vi "Destroy.vi"(0 "reference in":refnum<class "Devices Controller.lvclass">, 5 "error in (no error)":errorcluster) -> (14 "reference out":refnum<class "Devices Controller.lvclass">, 19 "error out":errorcluster)   [LabVIEW 2015, in "Devices Controller.lvclass"]
doc: "Destructor."
uses:
  Devices Controller.lvclass
  <vilib>/addons/_AddQ/G#Object/G#Object.lvclass
  APP/peapod_class/peapod.lvclass
  APP/fitmate_class/fitmate.lvclass
  APP/cpet_class/cpet.lvclass
  APP/bodpod_class/bodpod.lvclass
  APP/rmr_class/rmr.lvclass
  APP/k4b2_class/k4b2.lvclass
  APP/k5_class/k5.lvclass
  APP/bb-pft_class/bb-pft.lvclass
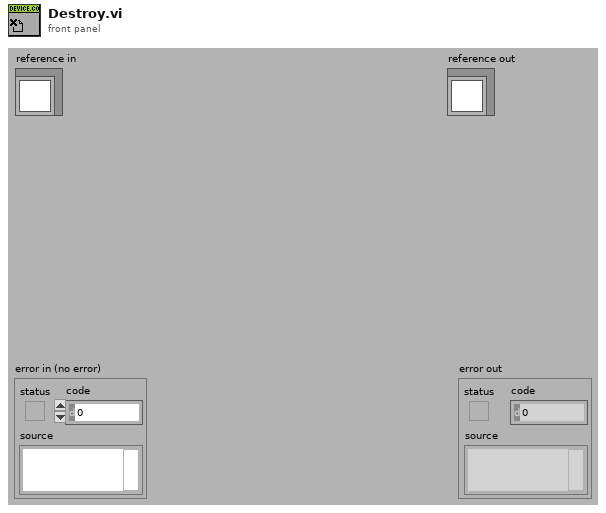
[diagram p1: front panel]
types:
  T1 = typedef "Devices Controller.lvclass/ObjectAttributes.ctl" = cluster{"MyAttribute":dbl, "file_controller_ref":refnum<class "File Controller.lvclass">, "data":string[][][], "devices_refs":cluster{"k4b2_refs":refnum<class "k4b2.lvclass">[], "rmr_refs":refnum<class "rmr.lvclass">[], "bod_pod_refs":refnum<class "bodpod.lvclass">[], "cpet_refs":refnum<class "cpet.lvclass">[], "fitmate_refs":refnum<class "fitmate.lvclass">[], "pea_pod_refs":refnum<class "peapod.lvclass">[], "k5_refs":refnum<class "k5.lvclass">[], "bb-pft_refs":refnum<class "bb-pft.lvclass">[]}}
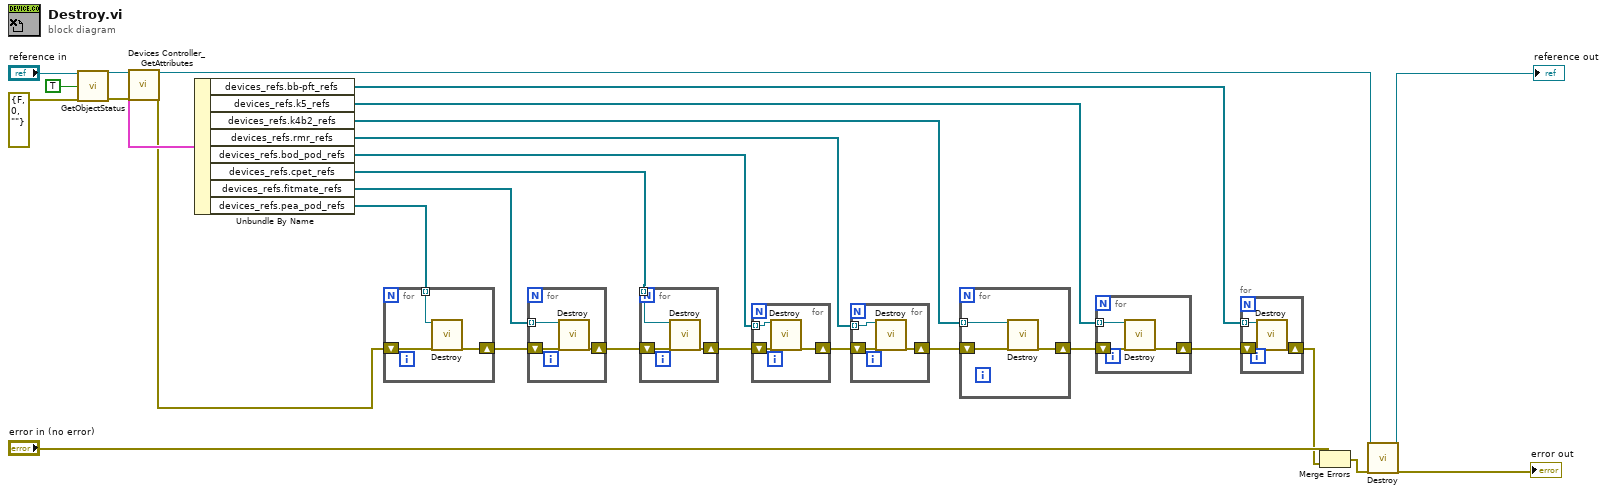
[diagram p0: block diagram]
diagram:
  n1 = call-dynamic "GetObjectStatus.vi"("reference in"="reference in", "simple info (F)"=TRUE ("simple info"), "error in (no error)"=errorcluster {"status"=FALSE, "code"=0, "source"=""}) -> ("reference out"=w22:refnum<class "Devices Controller.lvclass">, "error out"=w23:errorcluster)  [unwired: 5 in, 10 out]
  n2 = call "Devices Controller_GetAttributes.vi"("reference in"=w22, "error in (no error)"=w23) -> ("reference out"=w21:refnum<class "Devices Controller.lvclass">, "attributes"=w20:T1, "error out"=w8:errorcluster)  [unwired: 14 in, 1 out]
  n3 = Unbundle By Name(w20) -> ("devices_refs.bb-pft_refs"=w1:refnum<class "bb-pft.lvclass">[], "devices_refs.k5_refs"=w2:refnum<class "k5.lvclass">[], "devices_refs.k4b2_refs"=w17:refnum<class "k4b2.lvclass">[], "devices_refs.rmr_refs"=w15:refnum<class "rmr.lvclass">[], "devices_refs.bod_pod_refs"=w13:refnum<class "bodpod.lvclass">[], "devices_refs.cpet_refs"=w11:refnum<class "cpet.lvclass">[], "devices_refs.fitmate_refs"=w9:refnum<class "fitmate.lvclass">[], "devices_refs.pea_pod_refs"=w6:refnum<class "peapod.lvclass">[])
  n4 = for {
    tunnel: w6 -> [w29] mode=indexing
    shift-right: [w30] -> w7
    shift-left: w8 -> [w31]
    n5 = call-dynamic "Destroy.vi"("reference in"=w29, "error in (no error)"=w31) -> ("error out"=w30:errorcluster)  [unwired: 16 in, 1 out]
  }
  n6 = for {
    tunnel: w9 -> [w32] mode=indexing
    shift-right: [w33] -> w10
    shift-left: w7 -> [w34]
    n7 = call-dynamic "Destroy.vi"("reference in"=w32, "error in (no error)"=w34) -> ("error out"=w33:errorcluster)  [unwired: 16 in, 1 out]
  }
  n8 = for {
    tunnel: w11 -> [w35] mode=indexing
    shift-right: [w36] -> w12
    shift-left: w10 -> [w37]
    n9 = call-dynamic "Destroy.vi"("reference in"=w35, "error in (no error)"=w37) -> ("error out"=w36:errorcluster)  [unwired: 16 in, 1 out]
  }
  n10 = for {
    tunnel: w13 -> [w38] mode=indexing
    shift-right: [w39] -> w14
    shift-left: w12 -> [w40]
    n11 = call-dynamic "Destroy.vi"("reference in"=w38, "error in (no error)"=w40) -> ("error out"=w39:errorcluster)  [unwired: 16 in, 1 out]
  }
  n12 = for {
    tunnel: w15 -> [w41] mode=indexing
    shift-right: [w42] -> w16
    shift-left: w14 -> [w43]
    n13 = call-dynamic "Destroy.vi"("reference in"=w41, "error in (no error)"=w43) -> ("error out"=w42:errorcluster)  [unwired: 16 in, 1 out]
  }
  n14 = for {
    tunnel: w17 -> [w44] mode=indexing
    shift-right: [w45] -> w5
    shift-left: w16 -> [w46]
    n15 = call-dynamic "Destroy.vi"("reference in"=w44, "error in (no error)"=w46) -> ("error out"=w45:errorcluster)  [unwired: 16 in, 1 out]
  }
  n16 = for {
    tunnel: w2 -> [w47] mode=indexing
    shift-right: [w48] -> w4
    shift-left: w5 -> [w49]
    n17 = call-dynamic "Destroy.vi"("reference in"=w47, "error in (no error)"=w49) -> ("error out"=w48:errorcluster)  [unwired: 16 in, 1 out]
  }
  n18 = for {
    tunnel: w1 -> [w50] mode=indexing
    shift-right: [w51] -> w3
    shift-left: w4 -> [w52]
    n19 = call-dynamic "Destroy.vi"("reference in"=w50, "error in (no error)"=w52) -> ("error out"=w51:errorcluster)  [unwired: 16 in, 1 out]
  }
  n20 = Merge Errors("error in (no error)", w3) -> (w27:errorcluster)
  n21 = call-parent "Destroy.vi"("reference in"=w21, "error in (no error)"=w27) -> ("reference out"=→"reference out":refnum<class "Devices Controller.lvclass">, "error out"=→"error out":errorcluster)  [unwired: 16 in]
